vi "ReadPressureDAQ.vi"(9 "Reactor Selector":T1(ring)) -> (3 "Array":dbl[](array[numeric]))   [LabVIEW 2022 SP3]
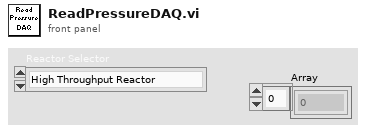
[diagram p1: front panel]
types:
  T1 = enum16{"High Throughput Reactor", "In Situ Reactor", "MLD Reactor"}
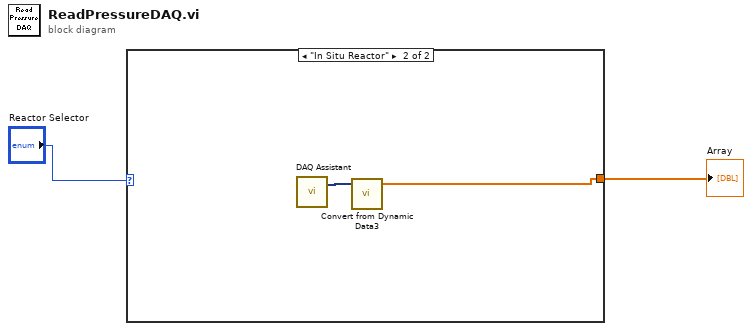
[diagram p0: block diagram]
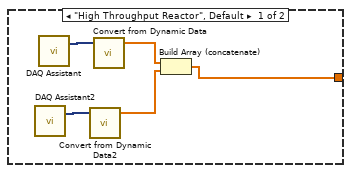
[diagram p2: hidden frame]
diagram:
  n1 = case shown="\"In Situ Reactor\"" "Reactor Selector" {
    tunnel: [w3 w8] -> w1
    frame "High Throughput Reactor", Default {
      n2 = call "DAQ Assistant2"() -> ("data"=w5:dynamicdata)  [unwired: 17 in, 2 out]
      n3 = call "DAQ Assistant"() -> ("data"=w4:dynamicdata)  [unwired: 17 in, 2 out]
      n4 = call "Convert from Dynamic Data2"("Dynamic Data Type"=w5) -> ("Array"=w7:dbl[])  [unwired: 3 in]
      n5 = call "Convert from Dynamic Data"("Dynamic Data Type"=w4) -> ("Array"=w6:dbl[])  [unwired: 3 in]
      n6 = Build Array (concatenate)(w6, w7) -> (w3:dbl[])
    }
    frame "In Situ Reactor" {
      n7 = call "DAQ Assistant"() -> ("data"=w9:dynamicdata)  [unwired: 17 in, 2 out]
      n8 = call "Convert from Dynamic Data3"("Dynamic Data Type"=w9) -> ("Array"=w8:dbl[])  [unwired: 3 in]
    }
  }
  "Array" <- w1
